vi "Start Pattern Core.vi"(8 "error in (no error)":errorcluster, 9 "Timeout":i32, 10 "Start Address":i32, 11 "CS++PPG in":refnum<class "CS++PPG.lvclass">) -> (0 "error out":errorcluster, 3 "CS++PPG out":refnum<class "CS++PPG.lvclass">)   [LabVIEW 2015, in "CS++PPG.lvlib" / "CS++PPG.lvclass"]
doc: "This VI starts the execution of the pattern (depending on the settings this could mean that the device first waits for an hardware trigger)."
uses:
  CS++PPG.lvclass
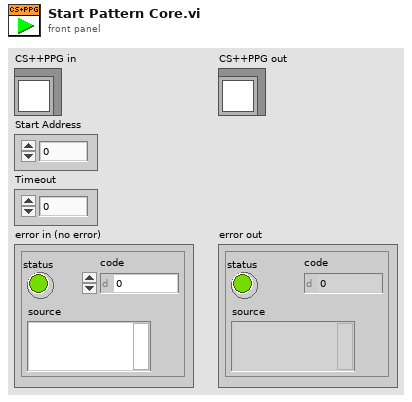
[diagram p1: front panel]
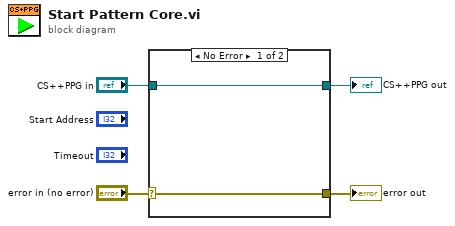
[diagram p0: block diagram]
diagram:
  n1 = case shown="No Error" "error in (no error)" {
    selector: "error in (no error)" -> [w5 w8]
    tunnel: [w5 w8] -> w3
    tunnel: [w6 w7] -> w1
    tunnel: "CS++PPG in" -> [w6 w7]
    frame No Error {
    }
    frame Error {
    }
  }
  "error out" <- w3
  "CS++PPG out" <- w1
